vi "1 axis move - Copy.vi"(1 "error in (no error)":errorcluster, 2 "Deceleration":bool, 5 "RESET":bool, 6 "Accelaration":bool, 7 "B axis":i32, 8 "Stop":bool, 9 "A axis":i32, 10 "Comport":refnum<visa-resource-name>) -> (3 "A out":dbl, 4 "B out":dbl)   [LabVIEW 2020]
uses:
  <vilib>/Instr/_visa.llb/VISA Configure Serial Port (Instr).vi
  GlobalValue.vi
panel:
  # "COMPORT"
  # "To Move"
  # "Moved"
  # "Microns"
  # "Microns"
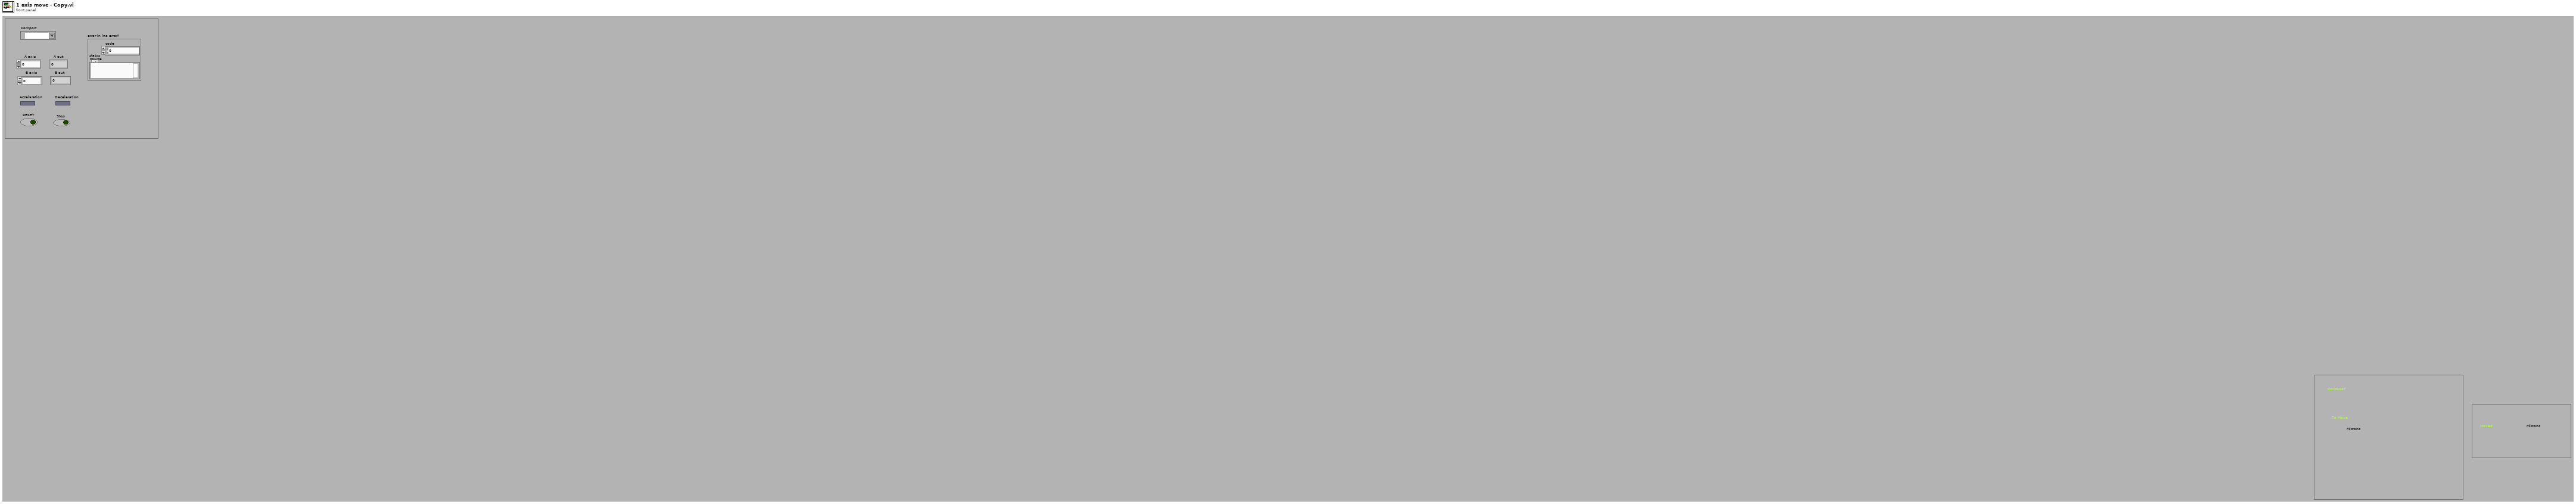
[diagram p1: front panel]
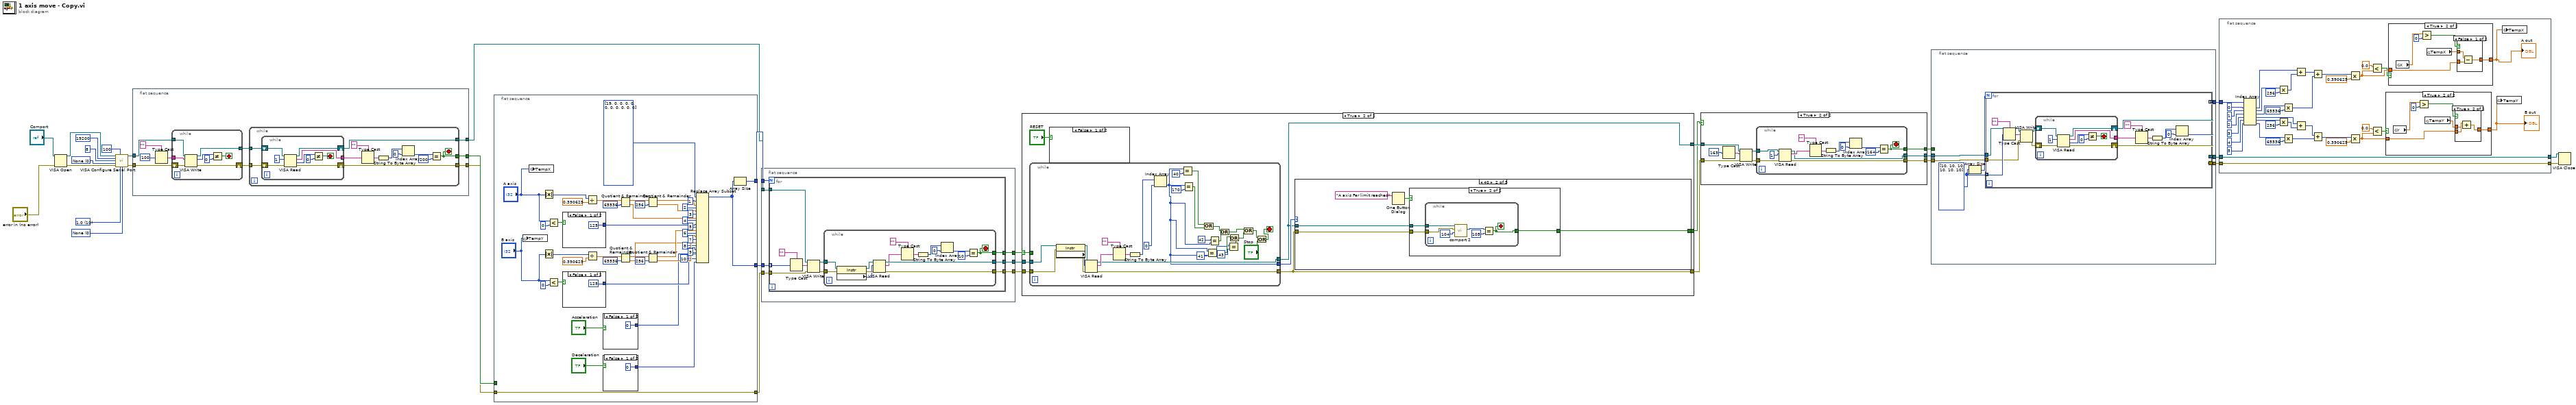
[diagram p0: block diagram]
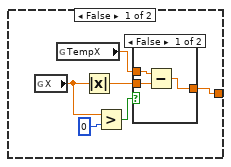
[diagram p2: hidden frame]
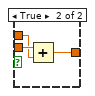
[diagram p3: hidden frame]
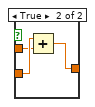
[diagram p4: hidden frame]
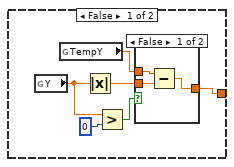
[diagram p5: hidden frame]
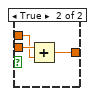
[diagram p6: hidden frame]
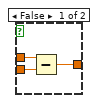
[diagram p7: hidden frame]
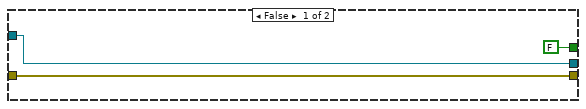
[diagram p8: hidden frame]
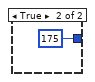
[diagram p9: hidden frame]
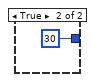
[diagram p10: hidden frame]
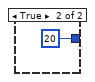
[diagram p11: hidden frame]
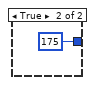
[diagram p12: hidden frame]
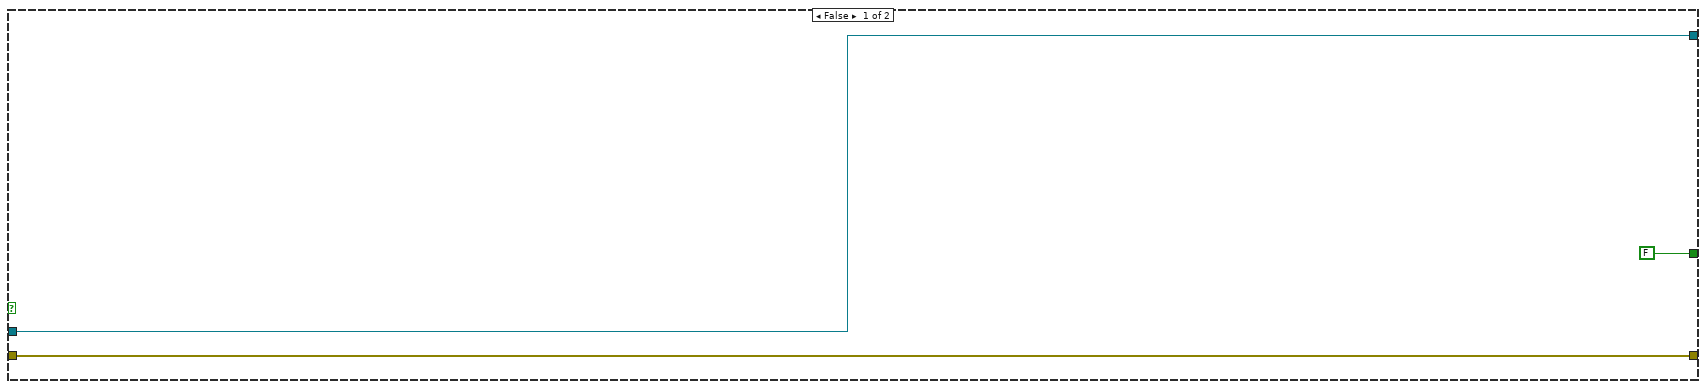
[diagram p13: hidden frame]
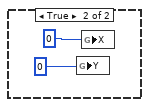
[diagram p14: hidden frame]
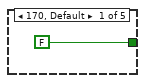
[diagram p15: hidden frame]
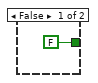
[diagram p16: hidden frame]
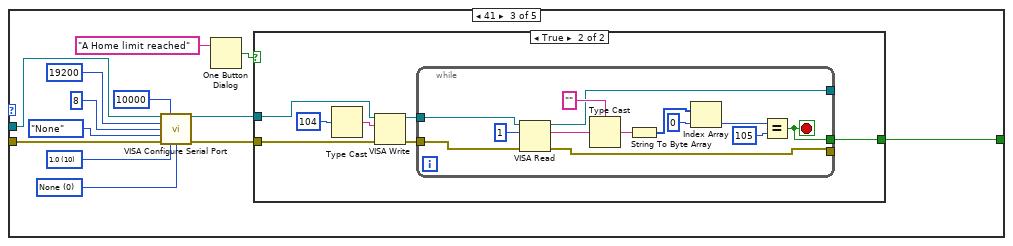
[diagram p17: hidden frame]
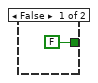
[diagram p18: hidden frame]
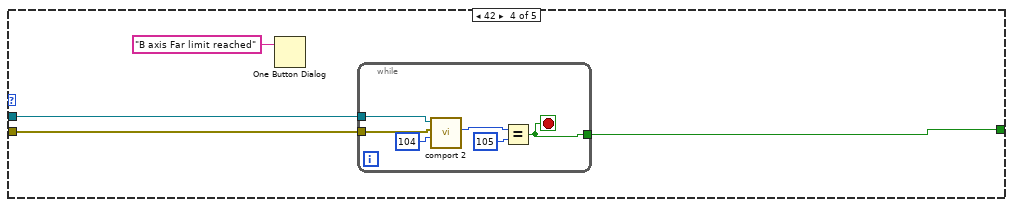
[diagram p19: hidden frame]
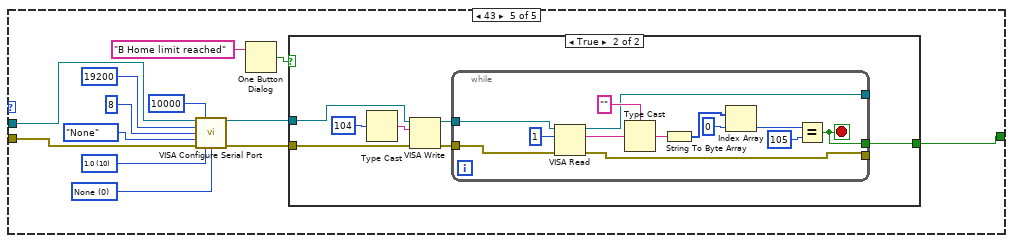
[diagram p20: hidden frame]
diagram:
  w27 = u16 0 items=["None"=0, "XON/XOFF"=1, "RTS/CTS"=2, "DTR/DSR"=4] ("flow control")
  w26 = u16 10 items=["1.0"=10, "1.5"=15, "2.0"=20] ("stop bits")
  w25 = u16 0 items=["None", "Odd", "Even", "Mark", "Space"] ("parity")
  n1 = VISA Open(error in (no error)="error in (no error)", VISA resource name="Comport") -> (VISA resource name=w30:refnum<visa-resource-name>, error out=w31:errorcluster)  [unwired: 3 in]
  n2 = call-poly "VISA Configure Serial Port"("VISA resource name"=w30, "timeout (10sec)"=u32 100, "baud rate (9600)"=u32 19200 ("baud rate"), "data bits (8)"=u16 8 ("data bits"), "parity (0:none)"=w25, "error in (no error)"=w31, "stop bits (10: 1 bit)"=w26, "flow control (0:none)"=w27) -> ("VISA resource name out"=w22:refnum<visa-resource-name>, "error out"=w21:errorcluster)  [unwired: 1 in, 5 out]
  n3 = flat-sequence {
    tunnel: w22 -> [w42]
    tunnel: w21 -> [w41]
    tunnel: [w40] -> w19
    tunnel: [w39] -> w6
    tunnel: [w33] -> w7
    frame #0 {
      n4 = Type Cast(type="", x=u8 100) -> (*(type *) &x=w37:string)
      n5 = while {
        tunnel: w37 -> [w50]
        shift-right: [w46] -> w34
        shift-left: w41 -> [w48]
        tunnel: w42 -> [w49]
        tunnel: [w47] -> w35
        stop <- w43 stop-if-true
        n6 = VISA Write(VISA resource name=w49, write buffer=w50, error in (no error)=w48) -> (VISA resource name out=w47:refnum<visa-resource-name>, return count=w45:u32, error out=w46:errorcluster)
        n7 = Not Equal?(x=w45, y=u32 0) -> (x != y?=w43:bool)
      }
      n8 = while {
        tunnel: w34 -> [w61]
        tunnel: [w59] -> w39
        tunnel: w35 -> [w62]
        tunnel: [w60] -> w40
        tunnel: [w54] -> w33
        stop <- w54 stop-if-true
        n9 = while {
          tunnel: [w66] -> w53
          shift-right: [w69] -> w60
          shift-left: w62 -> [w71]
          shift-right: [w68] -> w59
          shift-left: w61 -> [w70]
          stop <- w63 stop-if-true
          n10 = VISA Read(VISA resource name=w71, byte count=u32 1, error in (no error)=w70) -> (VISA resource name out=w69:refnum<visa-resource-name>, read buffer=w66:string, return count=w64:u32, error out=w68:errorcluster)
          n11 = Not Equal?(x=w64, y=u32 0) -> (x != y?=w63:bool)
        }
        n12 = Type Cast(type="", x=w53) -> (*(type *) &x=w51:string)
        n13 = String To Byte Array(string=w51) -> (unsigned byte array=w58:u8[])
        n14 = Index Array(array=w58, index=0) -> (element=w56:u8)
        n15 = Equal?(x=w56, y=u8 200) -> (x = y?=w54:bool)
      }
    }
  }
  n16 = flat-sequence {
    tunnel: [w110] -> w20
    tunnel: [w72] -> w18
    tunnel: w7 -> [_]
    tunnel: w6 -> [w107]
    tunnel: [w107] -> w5
    frame #0 {
      n17 = global write "GlobalValue.vi" "TempY"("B axis") -> ()
      n18 = global write "GlobalValue.vi" "TempX"("A axis") -> ()
      n19 = Absolute Value(x="A axis") -> (abs(x)=w111:i32)
      n20 = Absolute Value(x="B axis") -> (abs(x)=w99:i32)
      n21 = Less?(x="A axis", y=0) -> (x < y?=w113:bool)
      n22 = Less?(x="B axis", y=0) -> (x < y?=w94:bool)
      n23 = case shown="False" w113 {
        tunnel: [u16 125 u16 175] -> w85
        frame False {
        }
        frame True {
        }
      }
      n24 = case shown="False" w94 {
        tunnel: [u16 125 u16 175] -> w77
        frame False {
        }
        frame True {
        }
      }
      n25 = Divide(x=w111, y=0.390625) -> (x/y=w106:dbl)
      n26 = Divide(x=w99, y=0.390625) -> (x/y=w98:dbl)
      n27 = case shown="False" "Accelaration" {
        tunnel: [0 20] -> w75
        frame False {
        }
        frame True {
        }
      }
      n28 = case shown="False" "Deceleration" {
        tunnel: [0 30] -> w73
        frame False {
        }
        frame True {
        }
      }
      n29 = Quotient & Remainder(x=w106, y=65536) -> (x-y*floor(x/y)=w104:dbl, floor(x/y)=w88:dbl)
      n30 = Quotient & Remainder(x=w98, y=65536) -> (x-y*floor(x/y)=w96:dbl, floor(x/y)=w79:dbl)
      n31 = Quotient & Remainder(x=w104, y=256) -> (x-y*floor(x/y)=w91:dbl, floor(x/y)=w90:dbl)
      n32 = Quotient & Remainder(x=w96, y=256) -> (x-y*floor(x/y)=w83:dbl, floor(x/y)=w81:dbl)
      n33 = Replace Array Subset(array=u8[] [19, 0, 0, 0, 0, 0, 0, 0, 0, 0, 0], new element #1=w91, index #1=1 ("index"), new element #2=w90, index #2=2 ("index"), new element #3=w88, index #3=3 ("index"), new element #4=w85, index #4=4 ("index"), new element #5=w83, index #5=5 ("index"), new element #6=w81, index #6=6 ("index"), new element #7=w79, index #7=7 ("index"), new element #8=w77, index #8=8 ("index"), new element #9=w75, index #9=9 ("index"), new element #10=w73, index #10=10 ("index")) -> (w72:u8[])
      n34 = Array Size(array=w72) -> (size(s)=w110:i32)
    }
  }
  n35 = flat-sequence {
    tunnel: w20 -> [w130]
    tunnel: w19 -> [w129]
    tunnel: w5 -> [w128]
    tunnel: w18 -> [w127]
    tunnel: [w126] -> w17
    tunnel: [w125] -> w4
    tunnel: [w124] -> w16
    frame #0 {
      n36 = for {
        N: w130 -> [_]
        tunnel: [w135] -> w124
        tunnel: w129 -> [w139]
        tunnel: [w137] -> w126
        tunnel: w128 -> [w138]
        tunnel: [w136] -> w125
        tunnel: w127 -> [w132] mode=indexing
        n37 = Type Cast(type="", x=w132) -> (*(type *) &x=w131:string)
        n38 = VISA Write(VISA resource name=w139, write buffer=w131, error in (no error)=w138) -> (VISA resource name out=w134:refnum<visa-resource-name>, error out=w133:errorcluster)  [unwired: 1 out]
        n39 = while {
          tunnel: w133 -> [w144]
          tunnel: [w154] -> w136
          tunnel: w134 -> [w145]
          tunnel: [w155] -> w137
          tunnel: [w149] -> w135
          stop <- w149 stop-if-true
          n40 = property class="Instr"(reference=w145, error in=w144) -> (reference out=w143:refnum<visa-resource-name>, error out=w142:errorcluster, "Serial Settings:Number of Bytes at Serial Port"=w141:u32)
          n41 = VISA Read(VISA resource name=w143, byte count=w141, error in (no error)=w142) -> (VISA resource name out=w155:refnum<visa-resource-name>, read buffer=w148:string, error out=w154:errorcluster)  [unwired: 1 out]
          n42 = Type Cast(type="", x=w148) -> (*(type *) &x=w146:string)
          n43 = String To Byte Array(string=w146) -> (unsigned byte array=w153:u8[])
          n44 = Index Array(array=w153, index=0) -> (element=w151:u8)
          n45 = Equal?(x=w151, y=u8 10) -> (x = y?=w149:bool)
        }
      }
    }
  }
  n46 = case shown="True" w16 {
    selector: w16 -> [_ w159]
    tunnel: w17 -> [w158 w163]
    tunnel: w4 -> [w157 w165]
    tunnel: [w158 w162] -> w15
    tunnel: [w157 w161] -> w14
    tunnel: [FALSE w160] -> w1
    frame False {
    }
    frame True {
      n47 = while {
        tunnel: w165 -> [w181]
        tunnel: [w185] -> w162
        tunnel: [w187] -> w161
        tunnel: [w167] -> w164
        tunnel: w163 -> [w182]
        tunnel: w159 -> [_]
        stop <- w168 stop-if-true
        n48 = property class="Instr"(reference=w182, error in=w181) -> (reference out=w180:refnum<visa-resource-name>, error out=w179:errorcluster, "Serial Settings:Number of Bytes at Serial Port"=w178:u32)
        n49 = VISA Read(VISA resource name=w180, byte count=w178, error in (no error)=w179) -> (VISA resource name out=w185:refnum<visa-resource-name>, read buffer=w194:string, error out=w187:errorcluster)  [unwired: 1 out]
        n50 = Type Cast(type="", x=w194) -> (*(type *) &x=w195:string)
        n51 = String To Byte Array(string=w195) -> (unsigned byte array=w193:u8[])
        n52 = Index Array(array=w193, index=0) -> (element=w167:u8)
        n53 = Equal?(x=w167, y=u8 40) -> (x = y?=w184:bool)
        n54 = Equal?(x=w167, y=u8 170) -> (x = y?=w186:bool)
        n55 = Or(x=w184, y=w186) -> (x .or. y?=w175:bool)
        n56 = Equal?(x=w167, y=u8 41) -> (x = y?=w173:bool)
        n57 = Equal?(x=u8 42 ("y"), y=w167) -> (x = y?=w174:bool)
        n58 = Or(x=w175, y=w174) -> (x .or. y?=w183:bool)
        n59 = Equal?(x=w167, y=u8 43) -> (x = y?=w172:bool)
        n60 = Or(x=w173, y=w172) -> (x .or. y?=w171:bool)
        n61 = Or(x=w183, y=w171) -> (x .or. y?=w170:bool)
        n62 = Or(x=w170, y="Stop") -> (x .or. y?=w168:bool)
      }
      n63 = case shown="False" "RESET" {
        frame False {
        }
        frame True {
          n64 = global write "GlobalValue.vi" "Y"(0) -> ()
          n65 = global write "GlobalValue.vi" "X"(0) -> ()
        }
      }
      n66 = case shown="40" w164 {
        tunnel: w162 -> [_ w200 w223 w250 w260]
        tunnel: w161 -> [_ w201 w220 w249 w259]
        tunnel: [FALSE w199 w224 w248 w258] -> w160
        frame 170, Default {
        }
        frame 40 {
          n67 = One Button Dialog(message="A axis Far limit reached") -> (true=w202:bool)  [unwired: 1 in]
          n68 = case shown="True" w202 {
            tunnel: w201 -> [_ w206]
            tunnel: w200 -> [_ w207]
            tunnel: [FALSE w205] -> w199
            frame False {
            }
            frame True {
              n69 = while {
                tunnel: w207 -> [w213]
                tunnel: w206 -> [w212]
                tunnel: [w208] -> w205
                stop <- w208 stop-if-true
                n70 = call "comport 2.vi"("x"=u8 104, "error in (no error)"=w212, "VISA resource name"=w213) -> ("Numeric"=w210:u8)  [unwired: 6 in, 2 out]
                n71 = Equal?(x=w210, y=u8 105) -> (x = y?=w208:bool)
              }
            }
          }
        }
        frame 41 {
          w215 = u16 0 items=["None", "XON/XOFF", "RTS/CTS", "XON/XOFF & RTS/CTS", "DTR/DSR", "XON/XOFF & DTR/DSR"] ("flow control (0:none)")
          w216 = u16 10 items=["1.0"=10, "1.5"=15, "2.0"=20] ("stop bits (10: 1 bit)")
          n72 = call-poly "VISA Configure Serial Port"("VISA resource name"=w223, "timeout (10sec)"=u32 10000, "baud rate (9600)"=u32 19200, "data bits (8)"=u16 8, "parity (0:none)"=enum16{"None", "Odd", "Even", "Mark", "Space"}."None", "error in (no error)"=w220, "stop bits (10: 1 bit)"=w216, "flow control (0:none)"=w215) -> ("VISA resource name out"=w222:refnum<visa-resource-name>, "error out"=w221:errorcluster)  [unwired: 6 in]
          n73 = One Button Dialog(message="A Home limit reached") -> (true=w225:bool)  [unwired: 1 in]
          n74 = case shown="True" w225 {
            tunnel: w222 -> [_ w231]
            tunnel: w221 -> [_ w230]
            tunnel: [FALSE w228] -> w224
            frame False {
            }
            frame True {
              n75 = Type Cast(x=104) -> (*(type *) &x=w234:string)  [unwired: 1 in]
              n76 = VISA Write(VISA resource name=w231, write buffer=w234, error in (no error)=w230) -> (VISA resource name out=w232:refnum<visa-resource-name>, error out=w233:errorcluster)  [unwired: 1 out]
              n77 = while {
                tunnel: w233 -> [w247]
                tunnel: [w237] -> _
                tunnel: w232 -> [w246]
                tunnel: [w236] -> _
                tunnel: [w235] -> w228
                stop <- w235 stop-if-true
                n78 = VISA Read(VISA resource name=w246, byte count=u32 1, error in (no error)=w247) -> (VISA resource name out=w236:refnum<visa-resource-name>, read buffer=w238:string, error out=w237:errorcluster)  [unwired: 1 out]
                n79 = Type Cast(type="", x=w238) -> (*(type *) &x=w239:string)
                n80 = String To Byte Array(string=w239) -> (unsigned byte array=w243:u8[])
                n81 = Index Array(array=w243, index=0) -> (element=w240:u8)
                n82 = Equal?(x=w240, y=u8 105) -> (x = y?=w235:bool)
              }
            }
          }
        }
        frame 42 {
          n83 = One Button Dialog(message="B axis Far limit reached") -> ()  [unwired: 1 in, 1 out]
          n84 = while {
            tunnel: [w254] -> w248
            tunnel: w250 -> [w253]
            tunnel: w249 -> [w252]
            stop <- w254 stop-if-true
            n85 = call "comport 2.vi"("x"=u8 104, "error in (no error)"=w252, "VISA resource name"=w253) -> ("Numeric"=w256:u8)  [unwired: 6 in, 2 out]
            n86 = Equal?(x=w256, y=u8 105) -> (x = y?=w254:bool)
          }
        }
        frame 43 {
          w262 = u16 0 items=["None", "XON/XOFF", "RTS/CTS", "XON/XOFF & RTS/CTS", "DTR/DSR", "XON/XOFF & DTR/DSR"] ("flow control (0:none)")
          w263 = u16 10 items=["1.0"=10, "1.5"=15, "2.0"=20] ("stop bits (10: 1 bit)")
          n87 = call-poly "VISA Configure Serial Port"("VISA resource name"=w260, "timeout (10sec)"=u32 10000, "baud rate (9600)"=u32 19200, "data bits (8)"=u16 8, "parity (0:none)"=enum16{"None", "Odd", "Even", "Mark", "Space"}."None", "error in (no error)"=w259, "stop bits (10: 1 bit)"=w263, "flow control (0:none)"=w262) -> ("VISA resource name out"=w268:refnum<visa-resource-name>, "error out"=w267:errorcluster)  [unwired: 6 in]
          n88 = One Button Dialog(message="B Home limit reached") -> (true=w269:bool)  [unwired: 1 in]
          n89 = case shown="True" w269 {
            tunnel: w268 -> [_ w275]
            tunnel: w267 -> [_ w274]
            tunnel: [FALSE w272] -> w258
            frame False {
            }
            frame True {
              n90 = Type Cast(x=104) -> (*(type *) &x=w278:string)  [unwired: 1 in]
              n91 = VISA Write(VISA resource name=w275, write buffer=w278, error in (no error)=w274) -> (VISA resource name out=w276:refnum<visa-resource-name>, error out=w277:errorcluster)  [unwired: 1 out]
              n92 = while {
                tunnel: w277 -> [w291]
                tunnel: [w281] -> _
                tunnel: w276 -> [w290]
                tunnel: [w280] -> _
                tunnel: [w279] -> w272
                stop <- w279 stop-if-true
                n93 = VISA Read(VISA resource name=w290, byte count=u32 1, error in (no error)=w291) -> (VISA resource name out=w280:refnum<visa-resource-name>, read buffer=w282:string, error out=w281:errorcluster)  [unwired: 1 out]
                n94 = Type Cast(type="", x=w282) -> (*(type *) &x=w283:string)
                n95 = String To Byte Array(string=w283) -> (unsigned byte array=w287:u8[])
                n96 = Index Array(array=w287, index=0) -> (element=w284:u8)
                n97 = Equal?(x=w284, y=u8 105) -> (x = y?=w279:bool)
              }
            }
          }
        }
      }
    }
  }
  n98 = case shown="True" w1 {
    tunnel: w15 -> [w294 w300]
    tunnel: w14 -> [w293 w299]
    tunnel: [FALSE w298] -> w8
    tunnel: [w294 w296] -> w13
    tunnel: [w293 w297] -> w12
    frame False {
    }
    frame True {
      n99 = Type Cast(x=163) -> (*(type *) &x=w303:string)  [unwired: 1 in]
      n100 = VISA Write(VISA resource name=w300, write buffer=w303, error in (no error)=w299) -> (VISA resource name out=w301:refnum<visa-resource-name>, error out=w302:errorcluster)  [unwired: 1 out]
      n101 = while {
        tunnel: w302 -> [w316]
        tunnel: [w306] -> w297
        tunnel: w301 -> [w315]
        tunnel: [w305] -> w298
        tunnel: [w304] -> w296
        stop <- w305 stop-if-true
        n102 = VISA Read(VISA resource name=w315, byte count=u32 1, error in (no error)=w316) -> (VISA resource name out=w304:refnum<visa-resource-name>, read buffer=w307:string, error out=w306:errorcluster)  [unwired: 1 out]
        n103 = Type Cast(type="", x=w307) -> (*(type *) &x=w308:string)
        n104 = String To Byte Array(string=w308) -> (unsigned byte array=w312:u8[])
        n105 = Index Array(array=w312, index=0) -> (element=w309:u8)
        n106 = Equal?(x=w309, y=u8 164) -> (x = y?=w305:bool)
      }
    }
  }
  n107 = flat-sequence {
    tunnel: w12 -> [w322]
    tunnel: [w320] -> w10
    tunnel: [w321] -> w11
    tunnel: w13 -> [w319]
    tunnel: [w318] -> w9
    tunnel: w8 -> [_]
    frame #0 {
      w317 = u8[] [10, 10, 10, 10, 10, 10]
      n108 = Array Size(array=w317) -> (size(s)=w323:i32)
      n109 = for {
        N: w323 -> [_]
        tunnel: w322 -> [w326]
        tunnel: [w333] -> w321
        tunnel: w319 -> [w327]
        tunnel: [w332] -> w320
        tunnel: [w331] -> w318 mode=indexing
        tunnel: w317 -> [w328] mode=indexing
        n110 = Type Cast(type="", x=w328) -> (*(type *) &x=w329:string)
        n111 = VISA Write(VISA resource name=w327, write buffer=w329, error in (no error)=w326) -> (VISA resource name out=w325:refnum<visa-resource-name>, error out=w324:errorcluster)  [unwired: 1 out]
        n112 = while {
          tunnel: [w342] -> w336
          shift-right: [w345] -> w333
          shift-left: w325 -> [w347]
          shift-right: [w344] -> w332
          shift-left: w324 -> [w346]
          stop <- w339 stop-if-true
          n113 = VISA Read(VISA resource name=w347, byte count=u32 1, error in (no error)=w346) -> (VISA resource name out=w345:refnum<visa-resource-name>, read buffer=w342:string, return count=w340:u32, error out=w344:errorcluster)
          n114 = Not Equal?(x=w340, y=u32 0) -> (x != y?=w339:bool)
        }
        n115 = Type Cast(type="", x=w336) -> (*(type *) &x=w334:string)
        n116 = String To Byte Array(string=w334) -> (unsigned byte array=w338:u8[])
        n117 = Index Array(array=w338, index=0) -> (element=w331:u8)
      }
    }
  }
  n118 = flat-sequence {
    tunnel: w11 -> [w353]
    tunnel: w10 -> [w352]
    tunnel: w9 -> [w384]
    tunnel: [w353] -> w3
    tunnel: [w352] -> w2
    frame #0 {
      n119 = Index Array(array=w384, index #1=0 ("index"), index #2=1 ("index"), index #3=2 ("index"), index #4=3 ("index"), index #5=4 ("index"), index #6=5 ("index")) -> (element #1=w374:u8, element #2=w361:u8, element #3=w360:u8, element #4=w356:u8, element #5=w355:u8, element #6=w354:u8)
      n120 = Multiply(x=w361, y=u16 256) -> (x*y=w380:u16)
      n121 = Multiply(x=w355, y=u16 256) -> (x*y=w370:u16)
      n122 = Multiply(x=w360, y=u32 65536) -> (x*y=w379:u32)
      n123 = Multiply(x=w354, y=u32 65536) -> (x*y=w369:u32)
      n124 = Add(x=w374, y=w380) -> (x+y=w378:u16)
      n125 = Add(x=w356, y=w370) -> (x+y=w368:u16)
      n126 = Add(x=w378, y=w379) -> (x+y=w376:u32)
      n127 = Add(x=w368, y=w369) -> (x+y=w364:u32)
      n128 = Multiply(x=w376, y=0.390625) -> (x*y=w351:dbl)
      n129 = Multiply(x=w364, y=0.390625) -> (x*y=w365:dbl)
      n130 = Less?(x=0.0, y=w351) -> (x < y?=w348:bool)
      n131 = Less?(x=0.0, y=w365) -> (x < y?=w366:bool)
      n132 = case shown="True" w366 {
        tunnel: w365 -> [_ w421]
        tunnel: [w411 w423] -> w349
        frame False {
          n133 = global read "GlobalValue.vi" "Y"() -> (w410:dbl)
          n134 = global read "GlobalValue.vi" "TempY"() -> (w412:dbl)
          n135 = Absolute Value(x=w410) -> (abs(x)=w409:dbl)
          n136 = Greater?(x=w410, y=0) -> (0:w413:bool)
          n137 = case shown="False" w413 {
            tunnel: w409 -> [w416 w420]
            tunnel: w412 -> [w417 w419]
            tunnel: [w415 w418] -> w411
            frame False {
              n138 = Subtract(x=w417, y=w416) -> (x-y=w415:dbl)
            }
            frame True {
              n139 = Add(x=w420, y=w419) -> (x+y=w418:dbl)
            }
          }
        }
        frame True {
          n140 = global read "GlobalValue.vi" "Y"() -> (w422:dbl)
          n141 = Greater?(x=w422, y=0) -> (0:w425:bool)
          n142 = global read "GlobalValue.vi" "TempY"() -> (w424:dbl)
          n143 = case shown="True" w425 {
            tunnel: w421 -> [w428 w432]
            tunnel: w424 -> [w429 w431]
            tunnel: [w427 w430] -> w423
            frame False {
              n144 = Subtract(x=w429, y=w428) -> (x-y=w427:dbl)
            }
            frame True {
              n145 = Add(x=w432, y=w431) -> (x+y=w430:dbl)
            }
          }
        }
      }
      "B out" <- w349
      n146 = case shown="True" w348 {
        tunnel: w351 -> [_ w397]
        tunnel: [w387 w399] -> w350
        frame False {
          n147 = global read "GlobalValue.vi" "X"() -> (w386:dbl)
          n148 = global read "GlobalValue.vi" "TempX"() -> (w388:dbl)
          n149 = Absolute Value(x=w386) -> (abs(x)=w385:dbl)
          n150 = Greater?(x=w386, y=0) -> (0:w389:bool)
          n151 = case shown="False" w389 {
            tunnel: w385 -> [w392 w396]
            tunnel: w388 -> [w393 w395]
            tunnel: [w391 w394] -> w387
            frame False {
              n152 = Subtract(x=w393, y=w392) -> (x-y=w391:dbl)
            }
            frame True {
              n153 = Add(x=w396, y=w395) -> (x+y=w394:dbl)
            }
          }
        }
        frame True {
          n154 = global read "GlobalValue.vi" "X"() -> (w398:dbl)
          n155 = Greater?(x=w398, y=0) -> (0:w401:bool)
          n156 = global read "GlobalValue.vi" "TempX"() -> (w400:dbl)
          n157 = case shown="False" w401 {
            tunnel: w397 -> [w404 w408]
            tunnel: w400 -> [w405 w407]
            tunnel: [w403 w406] -> w399
            frame False {
              n158 = Subtract(x=w405, y=w404) -> (x-y=w403:dbl)
            }
            frame True {
              n159 = Add(x=w408, y=w407) -> (x+y=w406:dbl)
            }
          }
        }
      }
      "A out" <- w350
      n160 = global write "GlobalValue.vi" "TempY"(w349) -> ()
      n161 = global write "GlobalValue.vi" "TempX"(w350) -> ()
    }
  }
  n162 = VISA Close(VISA resource name=w3, error in (no error)=w2) -> ()  [unwired: 1 out]
